vi "Set Vehicle Position from wash step.vi"(8 "error in (no error)":errorcluster, 10 "Car Wash Steps":T1, 11 "Car Wash Controller Actor in":refnum<class "Car Wash Controller Actor.lvclass">) -> (0 "error out":errorcluster, 3 "Car Wash Controller Actor out":refnum<class "Car Wash Controller Actor.lvclass">)   [LabVIEW 2019, in "Car Wash Controller Actor.lvlib" / "Car Wash Controller Actor.lvclass"]
uses:
  Car Wash Controller Actor.lvclass
  Sim Entry Console Actor/Sim Entry Console Actor/Wash steps selection -Buttons.ctl
  Car Wash Controller Actor.lvclass/Car Wash Controller Actor.ctl
  Vehicle Position Simulation/Vehicle Position Simulation Messages/Update Vehicle Position Simulation Msg/Update Vehicle Position Simulation Msg.lvclass/Update Vehicle Position Simulation Msg.ctl
  <vilib>/ActorFramework/Message Enqueuer/Message Enqueuer.lvclass/Message Enqueuer.ctl
  <vilib>/ActorFramework/Message Enqueuer/Enqueue.vi
  Vehicle Position Simulation/Vehicle Position Simulation Messages/Update Vehicle Position Simulation Msg/Update Vehicle Position Simulation Msg.lvclass
  C:/Program Files (x86)/National Instruments/LabVIEW 2019/vi.lib/ActorFramework/Message/Message.lvclass
  <vilib>/ActorFramework/Message Priority Queue/Priority Enqueue.vi
  Sim Entry Console Actor/Sim Entry Console Actor/Simulated Entry Console Actor.lvclass
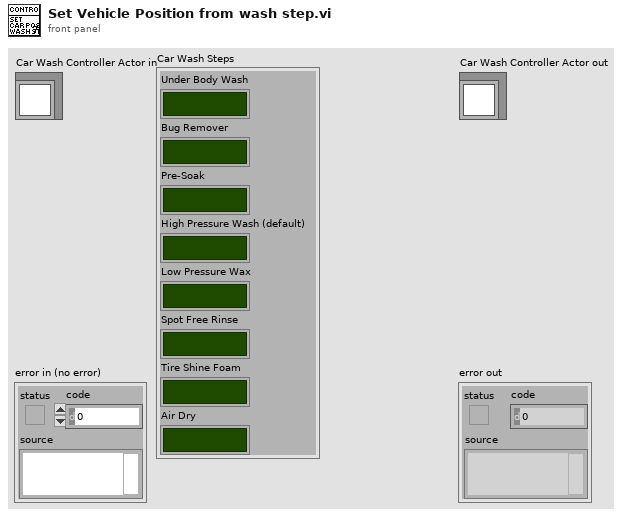
[diagram p1: front panel]
types:
  T1 = typedef "Simulated Entry Console Actor.lvlib/Simulated Entry Console Actor.lvclass/Wash steps selection -Buttons.ctl" = cluster{"Under Body Wash":bool, "Bug Remover":bool, "Pre-Soak":bool, "High Pressure Wash (default)":bool, "Low Pressure Wax":bool, "Spot Free Rinse":bool, "Tire Shine Foam":bool, "Air Dry":bool}
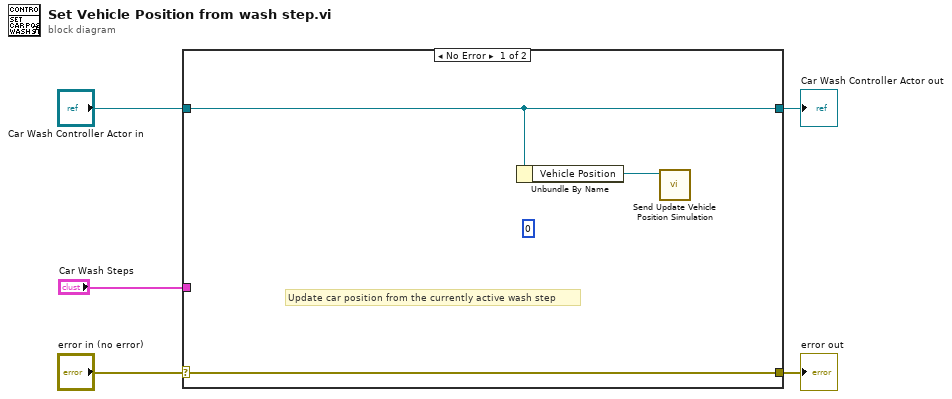
[diagram p0: block diagram]
diagram:
  n1 = case shown="No Error" "error in (no error)" {
    selector: "error in (no error)" -> [w8 w10]
    tunnel: [w8 w10] -> w4
    tunnel: [w7 w9] -> w2
    tunnel: "Car Wash Controller Actor in" -> [w7 w9]
    tunnel: "Car Wash Steps" -> [_ _]
    frame No Error {
      (unwired) u32 0 ("Vehicle Pos")
      # "Update car position from the currently active wash step"
      n2 = Unbundle By Name(w7) -> ("Vehicle Position"=w6:refnum<class "Message Enqueuer.lvclass">)
      n3 = call "Send Update Vehicle Position Simulation.vi"("Message Enqueuer"=w6) -> ()  [unwired: 9 in, 2 out]
    }
    frame Error {
    }
  }
  "error out" <- w4
  "Car Wash Controller Actor out" <- w2
